vi "TeleopSystem.vi"() -> ()   [LabVIEW 2025]
panel:
  out "SwerveDrive/GyroConnected":bool caption="Field Oriented"
  # "DRIVE"
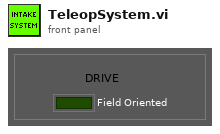
[diagram p1: front panel]
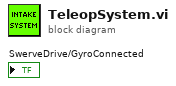
[diagram p0: block diagram]
diagram:
